vi "Load and Validate.vi"(8 "error in (no error)":errorcluster, 11 "Project Path":path) -> (0 "error out":errorcluster, 1 "Valid?":bool, 2 "Invalid Sections":string[](array[string]), 3 "Run cluster":T1)   [LabVIEW 2020, in "ProjectBuilder.lvlib"]
uses:
  ProjectBuilder.lvlib
  Ctl/Private/Ctl_Run Cluster.ctl
  Ctl/Ctl_Action Data.ctl
  Interface/Source Test/Source Test.lvclass
  Interface/Build/Build.lvclass
  Interface/Post-Build Test/Post-Build Test.lvclass
  Interface/Deploy/Deploy.lvclass
  Interface/Report Handler/Report Handler.lvclass
  Ctl/Private/Ctl_Build Steps.ctl
  PPL/HDH.ClassLoader.lvlibp
  <vilib>/Utility/config.llb/NI_LVConfig.lvlib
  <vilib>/Utility/Data Type/NI_Data Type.lvlib
  Interface/Project Action Interface/Project Action Interface.lvclass
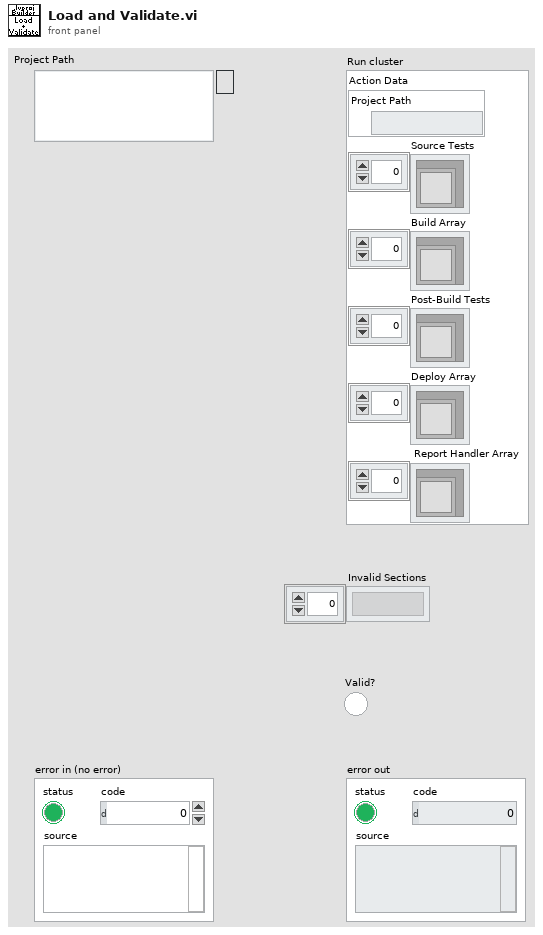
[diagram p1: front panel]
types:
  T1 = typedef "ProjectBuilder.lvlib/Ctl_Run Cluster.ctl" = cluster{"Action Data":T2, "Source Tests":refnum<class "Source Test.lvclass">[], "Build Array":refnum<class "Build.lvclass">[], "Post-Build Tests":refnum<class "Post-Build Test.lvclass">[], "Deploy Array":refnum<class "Deploy.lvclass">[], "Report Handler Array":refnum<class "Report Handler.lvclass">[]}
  T2 = typedef "ProjectBuilder.lvlib/Ctl_Action Data.ctl" = cluster{"Project Path":path}
  T3 = typedef "ProjectBuilder.lvlib/Ctl_Build Steps.ctl" = enum16{"Source Test", "Build", "Post-Build Test", "Deploy", "Report"}
  T4 = typedef "NI_LVConfig.lvlib/Config Data RefNum.ctl" = refnum<k1>
  T5 = cluster{"Build Step":T3, "Numeric":i32, "String":string}
  T6 = cluster{"Build Step":T3, "Numeric":i32, "String":string}[]
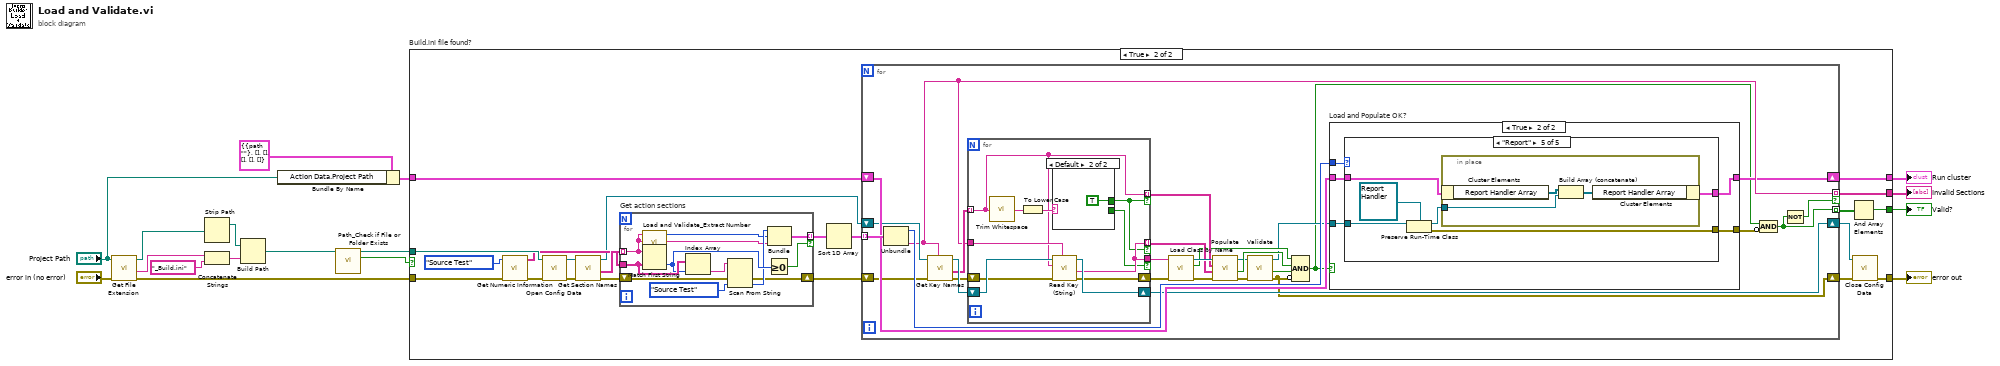
[diagram p0: block diagram]
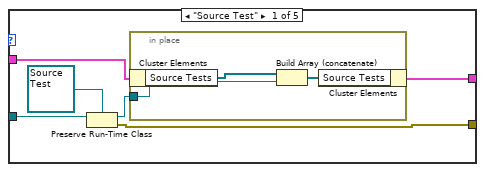
[diagram p4: hidden frame]
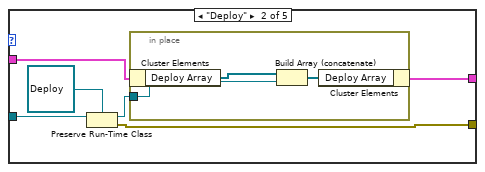
[diagram p5: hidden frame]
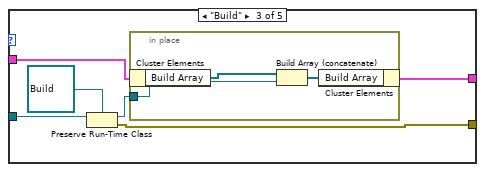
[diagram p6: hidden frame]
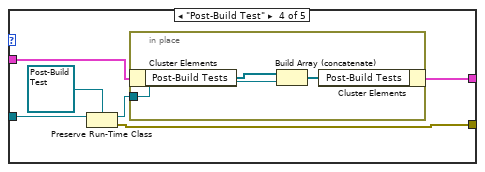
[diagram p7: hidden frame]
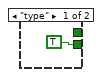
[diagram p8: hidden frame]
diagram:
  n1 = call <vilib>:"Get File Extension.vi"("error in (no error)"="error in (no error)", "file"="Project Path") -> ("error out"=w6:errorcluster, "filename without extension"=w15:string, "dup file"=w12:path)  [unwired: 5 in, 2 out]
  n2 = Strip Path(path=w12) -> (stripped path=w11:path)  [unwired: 1 out]
  n3 = Concatenate Strings(w15, "_Build.ini" ("string")) -> (w10:string)
  n4 = Build Path(base path=w11, name or relative path=w10) -> (appended path=w9:path)
  n5 = Bundle By Name(cluster=T1 {"Action Data"={"Project Path"=path ""}, "Source Tests"=[], "Build Array"=[], "Post-Build Tests"=[], "Deploy Array"=[], "Report Handler Array"=[]} ("Run Cluster"), "Action Data.Project Path"="Project Path") -> (w3:T1)
  n6 = call "Path_Check if File or Folder Exists.vi"("File or Folder Path in"=w9) -> ("File or Folder Found?"=w8:bool, "File or Folder Path dub"=w7:path)  [unwired: 9 in]
  n7 = case "Build.ini file found?" shown="True" w8 {
    tunnel: w7 -> [_ w40]
    tunnel: w6 -> [w19 w34]
    tunnel: [w19 w30] -> w5
    tunnel: [w18 w24] -> w4
    tunnel: w3 -> [w18 w23]
    tunnel: [_ w21] -> w2
    tunnel: [_ w20] -> w1
    frame False {
    }
    frame True {
      n8 = call <vilib>:"Get Numeric Information.vi"("error in (no error)"=w34, "variant"=Ctl_Build_Steps."Source Test" ("Build Step")) -> ("error out"=w33:errorcluster, "enum names"=w35:string[])  [unwired: 6 in, 2 out]
      n9 = call <vilib>:"Open Config Data.vi"("error in (no error)"=w33, "configuration file path"=w40) -> ("error out"=w38:errorcluster, "refnum"=w39:T4)  [unwired: 7 in, 1 out]
      n10 = call <vilib>:"Get Section Names.vi"("error in (no error)"=w38, "refnum"=w39) -> ("error out"=w32:errorcluster, "section names"=w37:string[], "refnum out"=w26:T4)  [unwired: 7 in]
      n11 = for "Get action sections" {
        tunnel: w37 -> [w133] mode=indexing
        tunnel: w35 -> [w143]
        shift-right: [w134] -> w28
        shift-left: w32 -> [w141]
        tunnel: [w140] -> w31 mode=indexing if=w139
        n12 = call "Load and Validate_Extract Number.vi"("String"=w133) -> ("Numeric"=w135:i32)  [unwired: 10 in]
        n13 = Match First String(2:w143, 3:w133) -> (0:w142:i32)  [unwired: 1 out]
        n14 = Index Array(array=w143, index=w142) -> (element=w138:string)
        n15 = Scan From String(input string=w138, error in=w141, default 1=Ctl_Build_Steps."Source Test" ("Build Step")) -> (error out=w134:errorcluster, output 1=w136:T3)  [unwired: 2 in, 2 out]
        n16 = Greater Or Equal To 0?(x=w142) -> (x >= 0?=w139:bool)
        n17 = Bundle("Build Step"=w136, "Numeric"=w135, "String"=w133) -> (w140:T5)  [unwired: 1 in]
      }
      n18 = Sort 1D Array(array=w31) -> (sorted array=w29:T6)
      n19 = for {
        tunnel: w29 -> [w68] mode=indexing
        shift-right: [w47] -> w27
        shift-left: w28 -> [w64]
        shift-right: [w62] -> w25
        shift-left: w26 -> [w65]
        shift-right: [w44] -> w24
        shift-left: w23 -> [w66]
        tunnel: [w41] -> w22 mode=indexing
        tunnel: [w46] -> w20 mode=indexing if=w45
        n20 = Unbundle(w68) -> ("Build Step"=w67:T3, "String"=w46:string)  [unwired: 1 out]
        n21 = call <vilib>:"Get Key Names.vi"("section"=w46, "error in (no error)"=w64, "refnum"=w65) -> ("error out"=w61:errorcluster, "key names"=w60:string[], "refnum out"=w63:T4)  [unwired: 5 in, 1 out]
        n22 = for {
          shift-right: [w129] -> w62
          shift-left: w63 -> [w130]
          shift-right: [w127] -> w58
          shift-left: w61 -> [w128]
          tunnel: w60 -> [w120] mode=indexing
          tunnel: w46 -> [w126]
          tunnel: [w125] -> w53 mode=indexing if=w122
          tunnel: [w120] -> w54 mode=indexing if=w122
          tunnel: [w125] -> w59 if=w121
          n23 = call <vilib>:"Trim Whitespace.vi"("string"=w120) -> ("trimmed string"=w124:string)  [unwired: 1 in]
          n24 = To Lower Case(string=w124) -> (all lower case string=w123:string)
          n25 = case shown="Default" w123 {
            tunnel: [_ TRUE] -> w122
            tunnel: [TRUE _] -> w121
            frame "type" {
            }
            frame Default {
            }
          }
          n26 = call <vilib>:"Read Key (String).vi"("section"=w126, "error in (no error)"=w128, "key"=w120, "refnum"=w130) -> ("error out"=w127:errorcluster, "value"=w125:string, "refnum out"=w129:T4)  [unwired: 4 in, 1 out]
        }
        n27 = call "Load Class by Name.vi"("error in (no error)"=w58, "Base Class Name"=w59) -> ("error out"=w57:errorcluster, "Class load Success?"=w52:bool, "Loaded Class"=w55:refnum<class>)  [unwired: 6 in, 1 out]
        n28 = call "Populate.vi"("error in (no error)"=w57, "Values"=w53, "Names"=w54, "Project Action Interface in"=w55) -> ("error out"=w56:errorcluster, "Success?"=w51:bool, "Project Action Interface out"=w50:refnum<class>)  [unwired: 5 in]
        n29 = call "Validate.vi"("error in (no error)"=w56, "Project Action Interface in"=w50) -> ("error out"=w47:errorcluster, "Valid?"=w48:bool, "Project Action Interface out"=w49:refnum<class>)  [unwired: 7 in]
        n30 = Compound Arithmetic op=AND(w52, w51, w48, invert w47) -> (w43:bool)
        n31 = case "Load and Populate OK?" shown="True" w43 {
          tunnel: w67 -> [_ w74]
          tunnel: w66 -> [w69 w73]
          tunnel: w49 -> [_ w72]
          tunnel: [w69 w71] -> w44
          tunnel: [_ w70] -> w42
          frame False {
          }
          frame True {
            n32 = case shown="\"Report\"" w74 {
              tunnel: w73 -> [w78 w87 w96 w105 w114]
              tunnel: w72 -> [w80 w89 w98 w107 w116]
              tunnel: [w76 w85 w94 w103 w112] -> w71
              tunnel: [w75 w84 w93 w102 w111] -> w70
              frame "Source Test" {
                n33 = Preserve Run-Time Class(object in=w80, 2:refnum<class "Source Test.lvclass"> refnum ("ProjectBuilder.lvlib:Source Test.lvclass")) -> (object out=w77:refnum<class "Source Test.lvclass">, error out=w75:errorcluster)  [unwired: 1 in]
                n34 = in-place {
                  in-place-border: w77 -> [w82]
                  n35 = in-place-cluster #1(w78) -> ("Source Tests"=w83:refnum<class "Source Test.lvclass">[])
                  n36 = Build Array (concatenate)(w83, w82) -> (w81:refnum<class "Source Test.lvclass">[])
                  n37 = in-place-cluster #1("Source Tests"=w81) -> (w76:T1)
                }
              }
              frame "Deploy" {
                n38 = Preserve Run-Time Class(object in=w89, 2:refnum<class "Deploy.lvclass"> refnum ("ProjectBuilder.lvlib:Deploy.lvclass")) -> (object out=w86:refnum<class "Deploy.lvclass">, error out=w84:errorcluster)  [unwired: 1 in]
                n39 = in-place {
                  in-place-border: w86 -> [w91]
                  n40 = in-place-cluster #2(w87) -> ("Deploy Array"=w92:refnum<class "Deploy.lvclass">[])
                  n41 = Build Array (concatenate)(w92, w91) -> (w90:refnum<class "Deploy.lvclass">[])
                  n42 = in-place-cluster #2("Deploy Array"=w90) -> (w85:T1)
                }
              }
              frame "Build" {
                n43 = Preserve Run-Time Class(object in=w98, 2:refnum<class "Build.lvclass"> refnum ("ProjectBuilder.lvlib:Build.lvclass")) -> (object out=w95:refnum<class "Build.lvclass">, error out=w93:errorcluster)  [unwired: 1 in]
                n44 = in-place {
                  in-place-border: w95 -> [w100]
                  n45 = in-place-cluster #3(w96) -> ("Build Array"=w101:refnum<class "Build.lvclass">[])
                  n46 = Build Array (concatenate)(w101, w100) -> (w99:refnum<class "Build.lvclass">[])
                  n47 = in-place-cluster #3("Build Array"=w99) -> (w94:T1)
                }
              }
              frame "Post-Build Test" {
                n48 = Preserve Run-Time Class(object in=w107, 2:refnum<class "Post-Build Test.lvclass"> refnum ("ProjectBuilder.lvlib:Post-Build Test.lvclass")) -> (object out=w104:refnum<class "Post-Build Test.lvclass">, error out=w102:errorcluster)  [unwired: 1 in]
                n49 = in-place {
                  in-place-border: w104 -> [w109]
                  n50 = in-place-cluster #4(w105) -> ("Post-Build Tests"=w110:refnum<class "Post-Build Test.lvclass">[])
                  n51 = Build Array (concatenate)(w110, w109) -> (w108:refnum<class "Post-Build Test.lvclass">[])
                  n52 = in-place-cluster #4("Post-Build Tests"=w108) -> (w103:T1)
                }
              }
              frame "Report" {
                n53 = Preserve Run-Time Class(object in=w116, 2:refnum<class "Report Handler.lvclass"> refnum ("ProjectBuilder.lvlib:Report Handler.lvclass")) -> (object out=w113:refnum<class "Report Handler.lvclass">, error out=w111:errorcluster)  [unwired: 1 in]
                n54 = in-place {
                  in-place-border: w113 -> [w118]
                  n55 = in-place-cluster #5(w114) -> ("Report Handler Array"=w119:refnum<class "Report Handler.lvclass">[])
                  n56 = Build Array (concatenate)(w119, w118) -> (w117:refnum<class "Report Handler.lvclass">[])
                  n57 = in-place-cluster #5("Report Handler Array"=w117) -> (w112:T1)
                }
              }
            }
          }
        }
        n58 = Compound Arithmetic op=AND(w43, invert w42) -> (w41:bool)
        n59 = Not(x=w41) -> (.not. x?=w45:bool)
      }
      n60 = And Array Elements(Boolean array=w22) -> (logical AND=w21:bool)
      n61 = call <vilib>:"Close Config Data.vi"("error in (no error)"=w27, "refnum"=w25) -> ("error out"=w30:errorcluster)  [unwired: 8 in, 1 out]
    }
  }
  "error out" <- w5
  "Run cluster" <- w4
  "Valid?" <- w2
  "Invalid Sections" <- w1
